vi "Configure Trigger (Delay).vi"(0 "VISA resource name":refnum<visa-resource-name>, 1 "Trigger Mode (0:Trigger After Time)":u16(ring) items=["Trigger After Time", "Trigger On nth Event"], 2 "Delay Time (30e-9)":dbl=3e-08, 3 "Event Number (0)":i32, 5 "Event Source (1: Channel 1)":u16(ring)=1 items=["Channel 1"=1, "Channel 2"=2, "Channel 3"=3, "Channel 4"=4, "Digital 0"=13, "Digital 1"=14, "Digital 2"=15, "Digital 3"=16, "Digital 4"=17, "Digital 5"=18, "Digital 6"=19, "Digital 7"=20, "Digital 8"=21, "Digital 9"=22, "Digital 10"=23, "Digital 11"=24, "Digital 12"=25, "Digital 13"=26, "Digital 14"=27, "Digital 15"=28], 7 "Event Slope (0: Positive)":u16(ring) items=["Positive", "Negative"], 9 "Event Level (0.0 V)":dbl, 11 "error in (no error)":errorcluster) -> (4 "VISA resource name out":refnum<visa-resource-name>, 15 "error out":errorcluster)   [LabVIEW 2012, in "Agilent 8000 Series.lvlib"]
doc: "Configures the delay trigger. It configures the Trigger Mode,Delay Time, Event Source and Slope, and the number of events to delay."
uses:
  <instrlib>/Agilent 8000 Series/Agilent 8000 Series.lvlib
panel:
  # "Trigger After Nth Event"
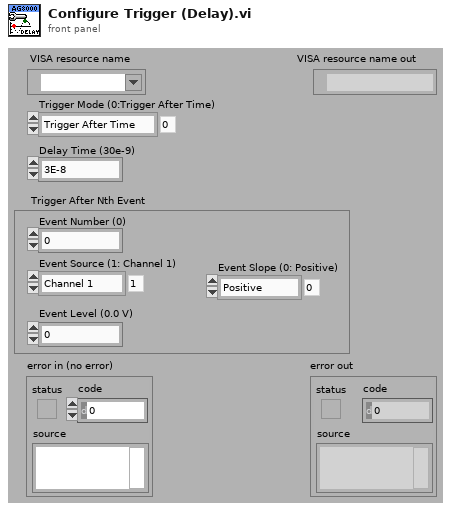
[diagram p1: front panel]
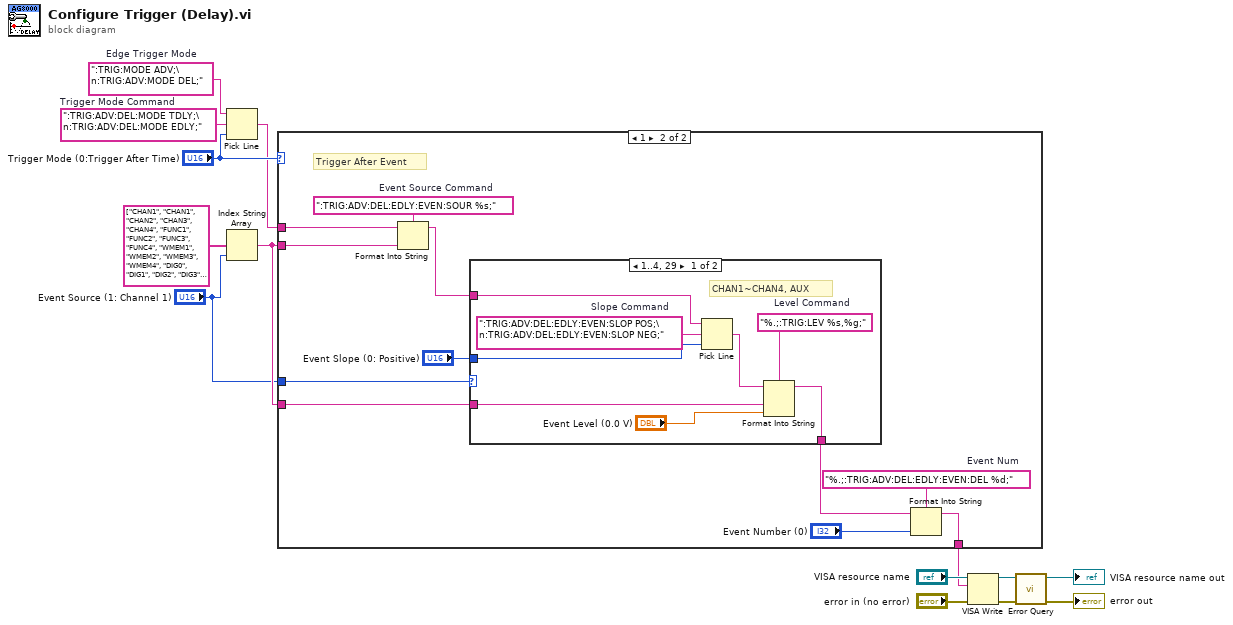
[diagram p0: block diagram]
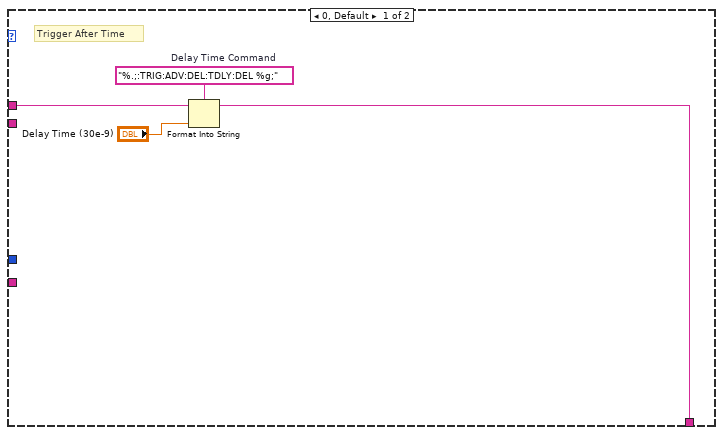
[diagram p2: hidden frame]
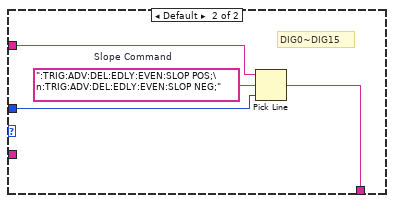
[diagram p3: hidden frame]
diagram:
  w8 = ":TRIG:ADV:DEL:MODE TDLY;\n:TRIG:ADV:DEL:MODE EDLY;"  # Trigger Mode Command
  w7 = ":TRIG:MODE ADV;\n:TRIG:ADV:MODE DEL;"  # Edge Trigger Mode
  n1 = Pick Line(string ("")=w7, multi-line string=w8, line index="Trigger Mode (0:Trigger After Time)") -> (output string=w5:string)
  n2 = Index String Array(1:"Event Source (1: Channel 1)", 2:string[] ["CHAN1", "CHAN1", "CHAN2", "CHAN3", "CHAN4", "FUNC1", "FUNC2", "FUNC3", "FUNC4", "WMEM1", "WMEM2", "WMEM3", "WMEM4", "DIG0", "DIG1", "DIG2", "DIG3", "DIG4", "DIG5", "DIG6", "DIG7", "DIG8", "DIG9", "DIG10", "DIG11", "DIG12", "DIG13", "DIG14", "DIG15", "AUX", "LINE"]) -> (0:w2:string)  [unwired: 1 in]
  n3 = case shown="1" "Trigger Mode (0:Trigger After Time)" {
    tunnel: w5 -> [w16 w24]
    tunnel: w2 -> [_ w28]
    tunnel: [w15 w25] -> w3
    tunnel: w2 -> [_ w20]
    tunnel: "Event Source (1: Channel 1)" -> [_ w19]
    frame 0, Default {
      w18 = "%.;:TRIG:ADV:DEL:TDLY:DEL %g;"  # Delay Time Command
      # "Trigger After Time"
      n4 = Format Into String(format string=w18, initial string=w16, "Delay Time (30e-9)") -> (resulting string=w15:string)  [unwired: 1 in, 1 out]
    }
    frame 1 {
      w27 = "%.;:TRIG:ADV:DEL:EDLY:EVEN:DEL %d;"  # Event Num
      w29 = ":TRIG:ADV:DEL:EDLY:EVEN:SOUR %s;"  # Event Source Command
      # "Trigger After Event"
      n5 = Format Into String(format string=w29, initial string=w24, w28) -> (resulting string=w21:string)  [unwired: 1 in, 1 out]
      n6 = case shown="1..4, 29" w19 {
        tunnel: [w36 w38] -> w22
        tunnel: "Event Slope (0: Positive)" -> [w34 w40]
        tunnel: w21 -> [w35 w39]
        tunnel: w20 -> [w32 _]
        frame 1..4, 29 {
          w31 = ":TRIG:ADV:DEL:EDLY:EVEN:SLOP POS;\n:TRIG:ADV:DEL:EDLY:EVEN:SLOP NEG;"  # Slope Command
          w37 = "%.;:TRIG:LEV %s,%g;"  # Level Command
          # "CHAN1~CHAN4, AUX"
          n7 = Pick Line(string ("")=w35, multi-line string=w31, line index=w34) -> (output string=w33:string)
          n8 = Format Into String(format string=w37, initial string=w33, w32, "Event Level (0.0 V)") -> (resulting string=w36:string)  [unwired: 1 in, 1 out]
        }
        frame Default {
          w41 = ":TRIG:ADV:DEL:EDLY:EVEN:SLOP POS;\n:TRIG:ADV:DEL:EDLY:EVEN:SLOP NEG;"  # Slope Command
          # "DIG0~DIG15"
          n9 = Pick Line(string ("")=w39, multi-line string=w41, line index=w40) -> (output string=w38:string)
        }
      }
      n10 = Format Into String(format string=w27, initial string=w22, "Event Number (0)") -> (resulting string=w25:string)  [unwired: 1 in, 1 out]
    }
  }
  n11 = VISA Write(VISA resource name="VISA resource name", write buffer=w3, error in (no error)="error in (no error)") -> (VISA resource name out=w10:refnum<visa-resource-name>, error out=w9:errorcluster)  [unwired: 1 out]
  n12 = call <instrlib>:"Error Query.vi"("error in (no error)"=w9, "VISA resource name"=w10) -> ("error out"=→"error out":errorcluster, "VISA resource name out"=→"VISA resource name out":refnum<visa-resource-name>)  [unwired: 6 in, 2 out]
